vi "Write Microscope Configuration.vi"(8 "error in (no error)":errorcluster, 10 "Microscope Configuration":T1={"Serial Port"="COM2", "Microscope Type"=enum."TE2000", "Detection Settings"=[]}, 11 "Ti2 in":refnum<class "Ti2.lvclass">) -> (0 "error out":errorcluster, 3 "Ti2 out":refnum<class "Ti2.lvclass">)   [LabVIEW 2018, in "Ti2.lvlib" / "Ti2.lvclass"]
uses:
  Ti2.lvclass
  Resources/Type Defs/Microscope Configuration.ctl
  Resources/Type Defs/Microscope Type.ctl
  Ti2.lvclass/Ti2.ctl
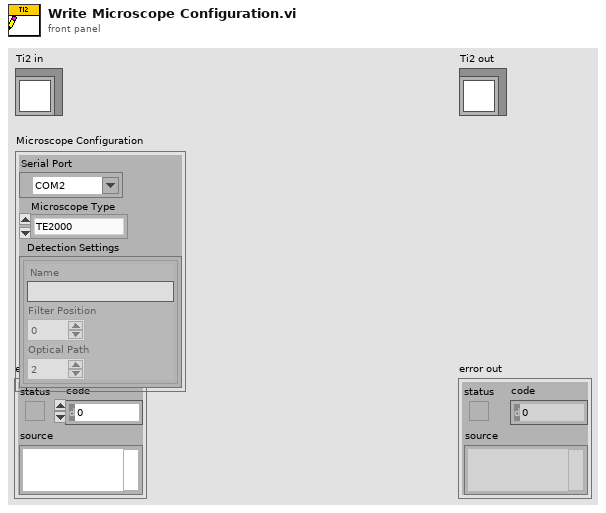
[diagram p1: front panel]
types:
  T1 = typedef "Microscope Configuration.ctl" = cluster{"Serial Port":refnum<visa-resource-name>, "Microscope Type":T2, "Detection Settings":cluster{"Name":string, "Filter Position":u16, "Optical Path":u16}[]}
  T2 = typedef "Microscope Type.ctl" = enum16{"Disable", "TE2000", "Eclipse Ti", "Ti2"}
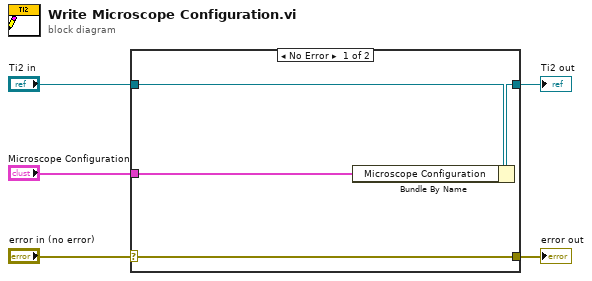
[diagram p0: block diagram]
diagram:
  n1 = case shown="No Error" "error in (no error)" {
    selector: "error in (no error)" -> [w9 w10]
    tunnel: [w9 w10] -> w4
    tunnel: [w7 w11] -> w2
    tunnel: "Ti2 in" -> [w8 w11]
    tunnel: "Microscope Configuration" -> [w6 _]
    frame No Error {
      n2 = Bundle By Name(cluster=w8, "Microscope Configuration"=w6) -> (w7:refnum<class "Ti2.lvclass">)
    }
    frame Error {
    }
  }
  "error out" <- w4
  "Ti2 out" <- w2
